vi "align_waveform.vi"(10 "Input Waveform":waveform(dbl), 11 "Sample Rate to be Wired":dbl) -> (3 "Output Waveform":waveform(dbl))   [LabVIEW 2019]
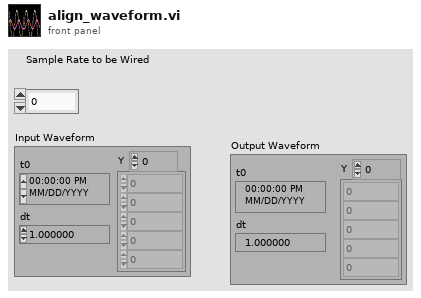
[diagram p1: front panel]
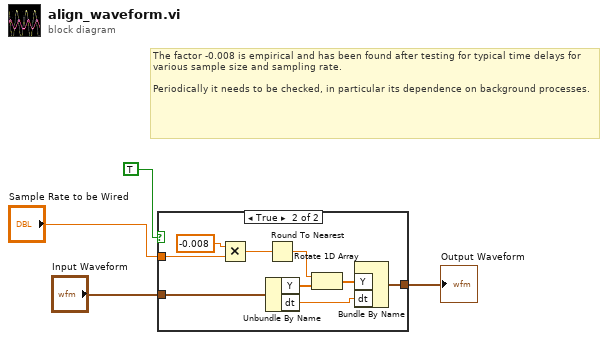
[diagram p0: block diagram]
diagram:
  # "The factor -0.008 is empirical and has been found after testing for typical time delays for various sample size and sampling rate.\n\nPeriodically it needs to be checked, in particular its dependence on background processes."
  n1 = case shown="True" TRUE ("Boolean") {
    tunnel: "Sample Rate to be Wired" -> [_ w14]
    tunnel: [w5 w11] -> w3
    tunnel: "Input Waveform" -> [w5 w10]
    frame False {
    }
    frame True {
      n2 = Multiply(x=-0.008, y=w14) -> (x*y=w12:dbl)
      n3 = Unbundle By Name(w10) -> ("Y"=w7:dbl[], "dt"=w9:dbl)
      n4 = Round To Nearest(number=w12) -> (nearest integer value=w13:dbl)
      n5 = Rotate 1D Array(1:w7, 2:w13) -> (0:w8:dbl[])
      n6 = Bundle By Name("Y"=w8, "dt"=w9) -> (w11:waveform(dbl))  [unwired: 1 in]
    }
  }
  "Output Waveform" <- w3
